vi "measurement.vi"(0 "Analog_Input.lvclass":refnum<class "Analog_Input.lvclass">, 11 "error in":errorcluster) -> (4 "AI Volts":dbl[](array[numeric]), 15 "error out":errorcluster)   [LabVIEW 2013, in "Analog_Input.lvclass"]
uses:
  Analog_Input.lvclass
  Analog_Input.lvclass/Analog_Input.ctl
  <vilib>/DAQmx/read.llb/DAQmx Read (Analog 1D Wfm NChan 1Samp).vi
  <vilib>/Analysis/baseanly.llb/Mean (DBL).vi
  Globals.vi
  <vilib>/DAQmx/miscellaneous.llb/DAQmx Fill In Error Info.vi
  <vilib>/Analysis/NI_AALBase.lvlib
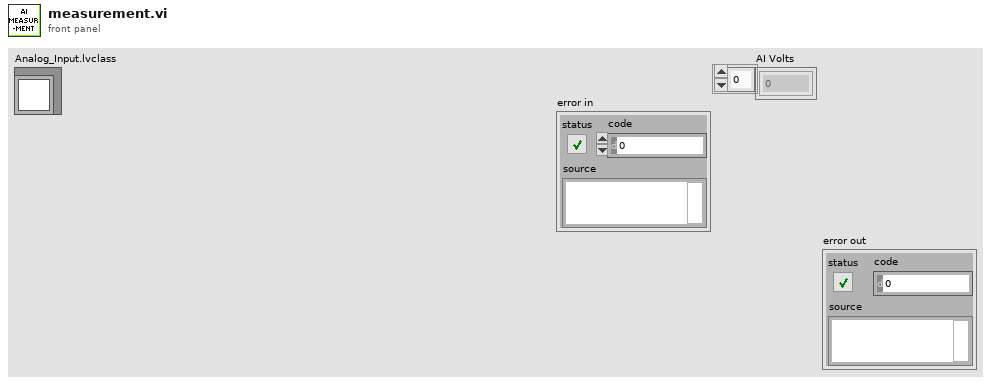
[diagram p1: front panel]
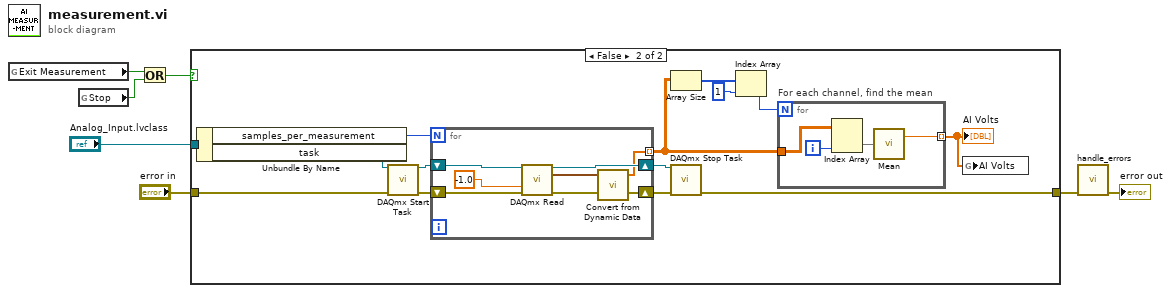
[diagram p0: block diagram]
diagram:
  n1 = global read "Globals.vi" "Exit Measurement"() -> (w4:bool)
  n2 = global read "Globals.vi" "Stop"() -> (w3:bool)
  n3 = Or(x=w4, y=w3) -> (x .or. y?=w2:bool)
  n4 = case shown="False" w2 {
    tunnel: "error in" -> [w8 w9]
    tunnel: [w8 w13] -> w6
    tunnel: "Analog_Input.lvclass" -> [_ w12]
    frame True {
    }
    frame False {
      n5 = Unbundle By Name(w12) -> ("samples_per_measurement"=w11:i32, "task"=w10:refnum<k21>)
      n6 = call <vilib>:"DAQmx Start Task.vi"("task/channels in"=w10, "error in"=w9) -> ("task out"=w21:refnum<k21>, "error out"=w22:errorcluster)  [unwired: 12 in]
      n7 = for {
        N: w11 -> [_]
        shift-right: [w29] -> w19
        shift-left: w21 -> [w30]
        shift-right: [w28] -> w20
        shift-left: w22 -> [w31]
        tunnel: [w27] -> w18 mode=indexing
        n8 = call-poly <vilib>:"DAQmx Read.vi"("task/channels in"=w30, "timeout"=-1.0, "error in"=w31) -> ("task out"=w29:refnum<k21>, "data"=w32:waveform(dbl)[], "error out"=w28:errorcluster)  [unwired: 10 in]
        n9 = call "Convert from Dynamic Data"("Dynamic Data Type"=w32) -> ("Array"=w27:dbl[])  [unwired: 3 in]
      }
      n10 = Array Size(array=w18) -> (size(s)=w17:i32[])
      n11 = call <vilib>:"DAQmx Stop Task.vi"("task/channels in"=w19, "error in"=w20) -> ("error out"=w13:errorcluster)  [unwired: 12 in, 1 out]
      n12 = Index Array(array=w17, index=1) -> (element=w15:i32)
      n13 = for "For each channel, find the mean" {
        N: w15 -> [_]
        tunnel: w18 -> [w26]
        tunnel: [w23] -> w14 mode=indexing
        i -> [w25]
        n14 = Index Array(array=w26, index (col)=w25) -> (element=w24:dbl[])  [unwired: 1 in]
        n15 = call-poly <vilib>:"Mean.vi"("X"=w24) -> ("mean"=w23:dbl)  [unwired: 1 out]
      }
      "AI Volts" <- w14
      n16 = global write "Globals.vi" "AI Volts"(w14) -> ()
    }
  }
  n17 = call "handle_errors.vi"("error in (no error)"=w6) -> ("error out"=→"error out":errorcluster)  [unwired: 14 in]
